vi "Ustaw konfig kanalow.vi"(8 "error in (no error)":errorcluster, 11 "Array":refnum<vi>[](array[refnum])) -> (0 "error out":errorcluster)   [LabVIEW 2014]
doc: "W zakładce Konfiguracja ustawia tab kanałów\ni przyciski\nustawienie na szywno wg tablicy podanej wewnątrz"
uses:
  <vilib>/Utility/miscctls.llb/LVPositionTypeDef.ctl
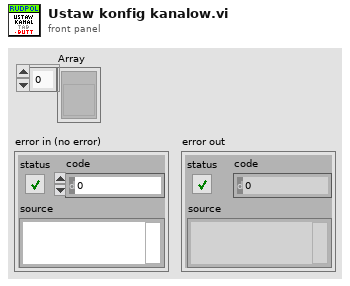
[diagram p1: front panel]
types:
  T1 = typedef "LVPositionTypeDef.ctl" = cluster{"Left":i32, "Top":i32}
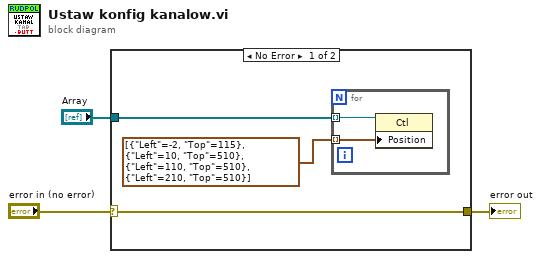
[diagram p0: block diagram]
diagram:
  n1 = case shown="No Error" "error in (no error)" {
    selector: "error in (no error)" -> [w4 w9]
    tunnel: "Array" -> [w5 _]
    tunnel: [w4 w9] -> w1
    frame No Error {
      n2 = for {
        tunnel: w5 -> [w8] mode=indexing
        tunnel: T1[] [{"Left"=-2, "Top"=115}, {"Left"=10, "Top"=510}, {"Left"=110, "Top"=510}, {"Left"=210, "Top"=510}] -> [w7] mode=indexing
        n3 = property class="Ctl"(reference=w8, "Position"=w7) -> ()  [unwired: 1 in, 2 out]
      }
    }
    frame Error {
    }
  }
  "error out" <- w1
